vi "Get LTS Max Stage Velocity and Acceleration_2.vi"(8 "error in (no error)":errorcluster, 10 "Cluster in":T1, 11 "LTS Reference In":refnum<k24>) -> (0 "error out":errorcluster, 2 "Cluster out":T1, 3 "LTS Reference Out":refnum<k24>)   [LabVIEW 2018]
uses:
  Controls/Translation Stage Cluster.ctl
  General/Controls/Translation Stage Types.ctl
  C:/Project/SerialSectOCT - FFT GPU/SerialSectOCT/Labview Software/Thorlabs.MotionControl.Controls.dll
  Thorlabs.MotionControl.Controls.dll
  C:/Project/SerialSectOCT - FFT GPU/SerialSectOCT/Labview Software/Thorlabs.MotionControl.IntegratedStepperMotorsCLI.dll
  Thorlabs.MotionControl.IntegratedStepperMotorsCLI.dll
  C:/Project/SerialSectOCT - FFT GPU/SerialSectOCT/Labview Software/Thorlabs.MotionControl.GenericMotorCLI.dll
  Thorlabs.MotionControl.GenericMotorCLI.dll
panel:
  out "Cluster Out":T1={"Position"=0.0, "Is.Enabled?"=FALSE, "Is.Connected?"=FALSE, "Device SN"="45876539", "AccelerationMaximum"=0.0, "VelocityMaximum"=0.0, "Acceleration"=0.0, "Velocity"=0.0, "waitTimeout (ms)"=0, "Model"=enum."None", "Is.Homed?"=FALSE}
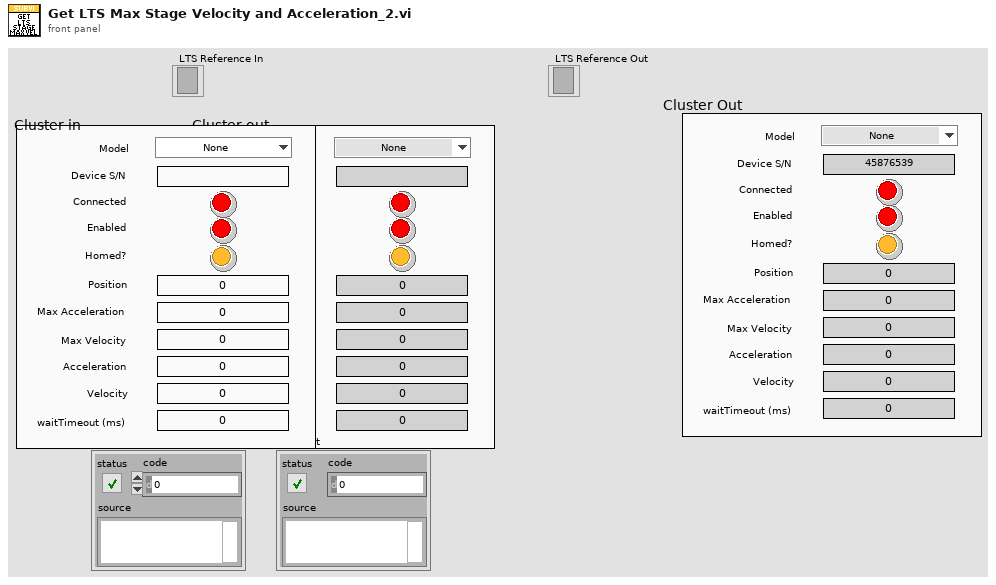
[diagram p1: front panel]
types:
  T1 = typedef "Translation Stage Cluster.ctl" = cluster{"Position":dbl, "Is.Enabled?":bool, "Is.Connected?":bool, "Device SN":string, "AccelerationMaximum":dbl, "VelocityMaximum":dbl, "Acceleration":dbl, "Velocity":dbl, "waitTimeout (ms)":i32, "Model":T2, "Is.Homed?":bool}
  T2 = typedef "Translation Stage Types.ctl" = enum16{"None", "Thorlabs LTS", "Thorlabs MLJ"}
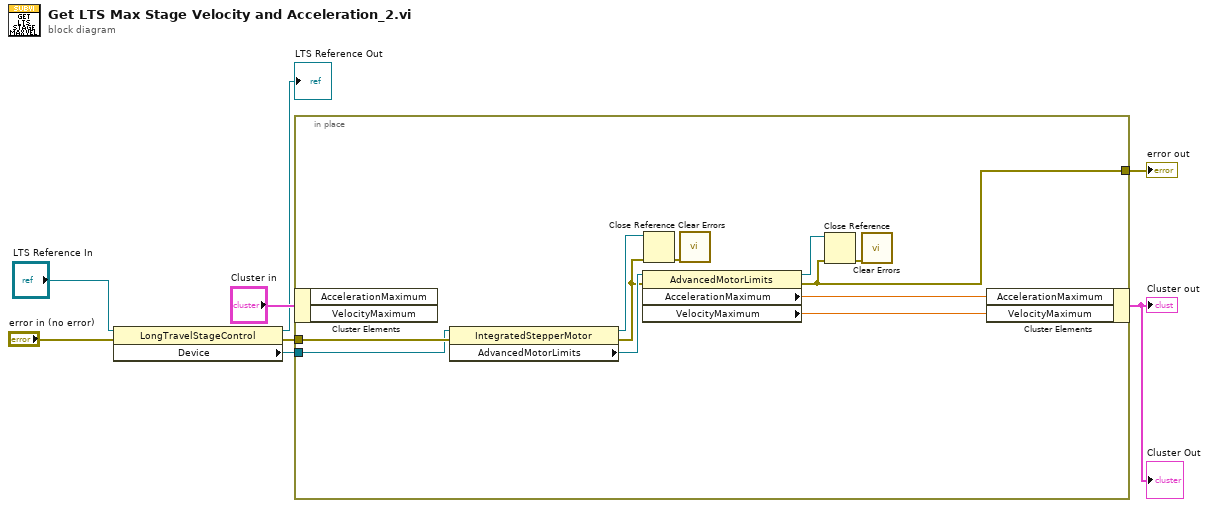
[diagram p0: block diagram]
diagram:
  n1 = property class="LongTravelStageControl"(reference="LTS Reference In", error in="error in (no error)") -> (reference out=→"LTS Reference Out":refnum<k24>, error out=w3:errorcluster, "Device"=w1:refnum<k24>)
  n2 = in-place {
    in-place-border: w3 -> [w19]
    in-place-border: [w10] -> w6
    in-place-border: w1 -> [w16]
    n3 = in-place-cluster #1("Cluster in") -> ()  [unwired: 2 out]
    n4 = property class="IntegratedStepperMotor"(reference=w16, error in=w19) -> (reference out=w17:refnum<k24>, error out=w9:errorcluster, "AdvancedMotorLimits"=w14:refnum<k24>)
    n5 = property class="AdvancedMotorLimits"(reference=w14, error in=w9) -> (reference out=w15:refnum<k24>, error out=w10:errorcluster, "AccelerationMaximum"=w13:dbl, "VelocityMaximum"=w12:dbl)
    n6 = Close Reference(reference=w17, error in (no error)=w9) -> (error out=w18:errorcluster)
    n7 = call <vilib>:"Clear Errors.vi"("error in (no error)"=w18) -> ()  [unwired: 5 in, 2 out]
    n8 = Close Reference(reference=w15, error in (no error)=w10) -> (error out=w11:errorcluster)
    n9 = call <vilib>:"Clear Errors.vi"("error in (no error)"=w11) -> ()  [unwired: 5 in, 2 out]
    n10 = in-place-cluster #1("AccelerationMaximum"=w13, "VelocityMaximum"=w12) -> (→"Cluster out" →"Cluster Out":T1)
  }
  "error out" <- w6
